vi "Test.vi"(0 "Traverse Algorithm in":refnum<class "Node Test.lvclass">, 5 "Terminal To Identify":refnum<vi>, 11 "error in (no error)":errorcluster) -> (4 "Traverse Algorithm out":refnum<class "Node Test.lvclass">, 6 "Terminal for Traversal Continuation":refnum<vi>[](array[refnum]), 8 "Node Identified":bool, 15 "error out":errorcluster)   [LabVIEW 2020, in "MVA Message Mapper.lvlib" / "Node Test.lvclass"]
uses:
  <vilib>/gpm_packages/@cs/Bus-message-mapper/Source/support/Traversal Algorithm/Node Test.lvclass
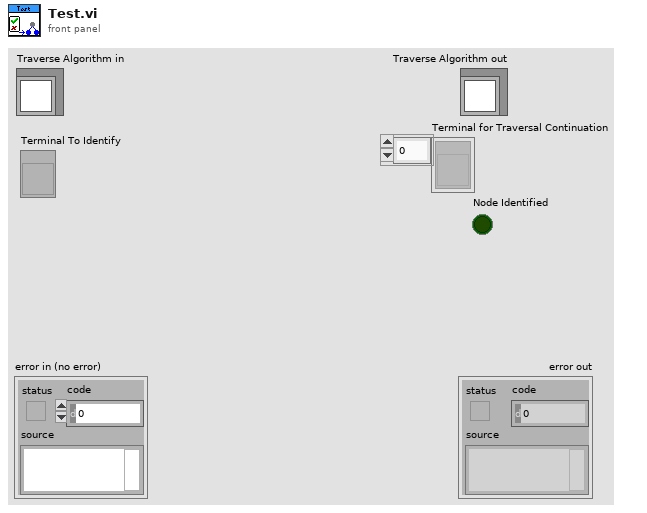
[diagram p1: front panel]
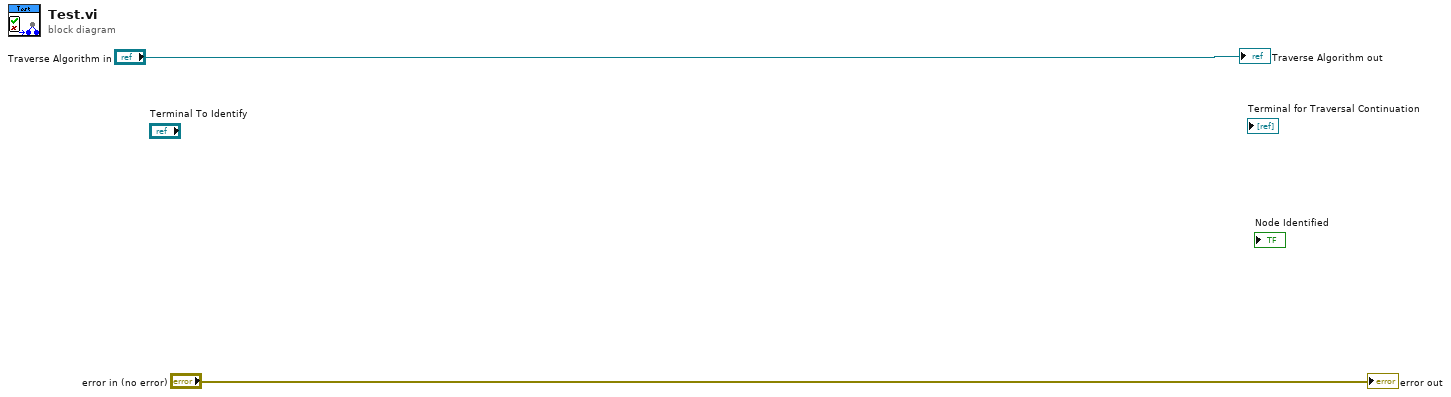
[diagram p0: block diagram]
diagram:
  "error out" <- "error in (no error)"
  "Traverse Algorithm out" <- "Traverse Algorithm in"
